vi "Filter Clusters Target.vi"() -> ()   [LabVIEW 2017]
panel:
  in  "Control":T1
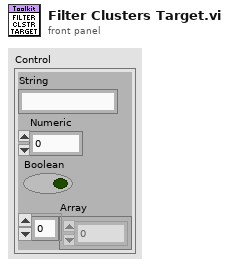
[diagram p1: front panel]
types:
  T1 = cluster{"String":string, "Numeric":dbl, "Boolean":bool, "Array":dbl[]}
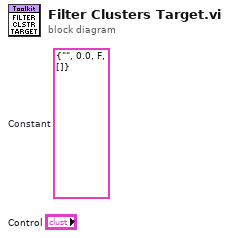
[diagram p0: block diagram]
diagram:
  (unwired) T1 {"String"="", "Numeric"=0.0, "Boolean"=FALSE, "Array"=[]}  # Constant
